vi "public_device_list.vi"() -> ()   [LabVIEW 2020]
panel:
  in  "public_device_list":string[](array[string])
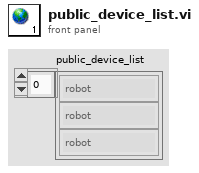
[diagram p1: front panel]
diagram:
